vi "Conversion.vi"(0 "read buffer":string, 9 "Mechanical Zero":dbl) -> (3 "Static LF":dbl, 4 "Dynamic LF":dbl, 6 "Dynamic Load Force":dynamicdata(graph), 8 "Elbow Angle (deg)":dbl, 10 "GF":dbl, 13 "Static Load Force":dynamicdata(graph), 14 "Grip Force":dynamicdata(graph), 15 "Goniometer\nAngle Raw":dynamicdata(graph))   [LabVIEW 2018]
doc: "VI for GF and LF conversion."
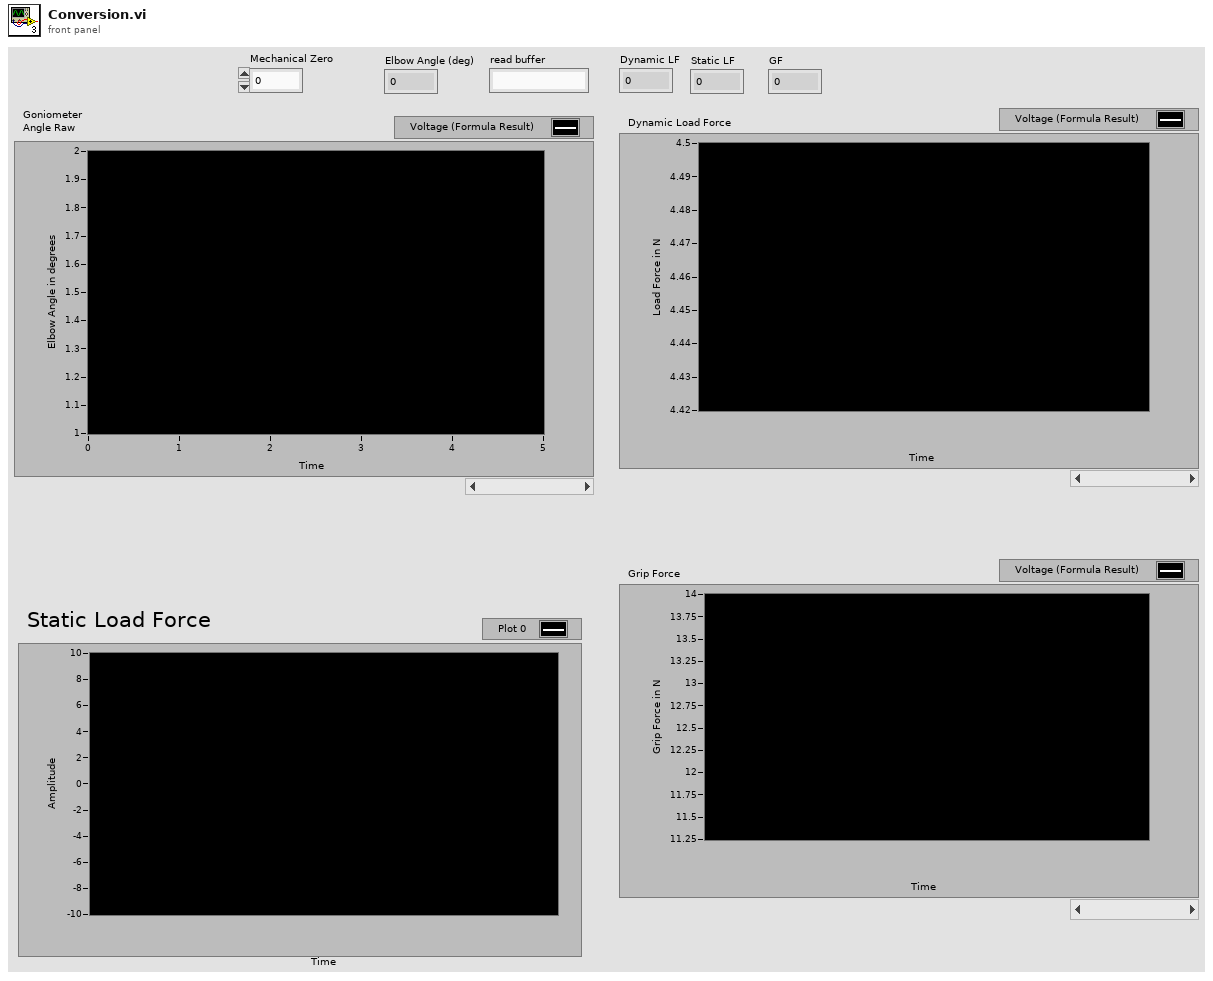
[diagram p1: front panel]
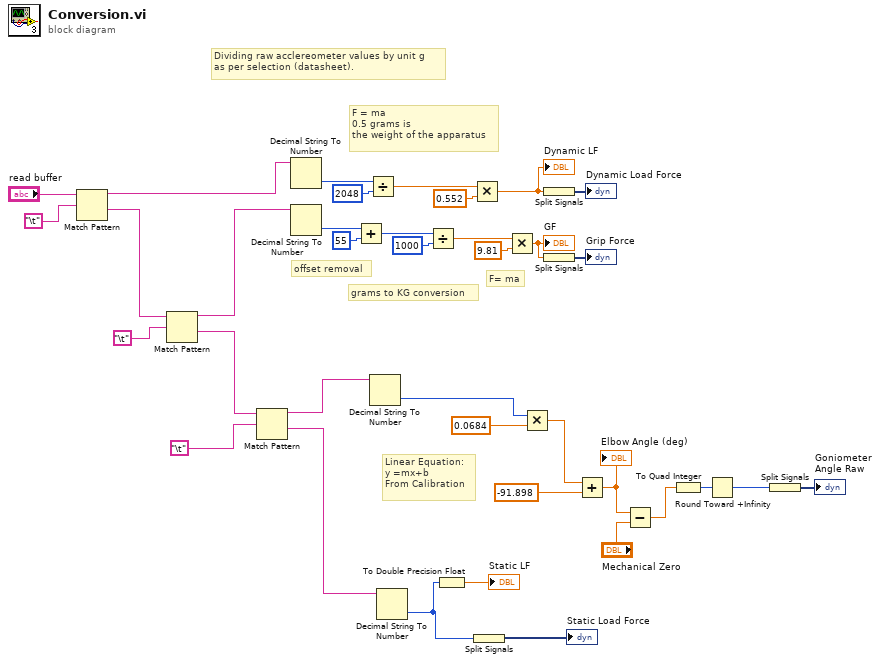
[diagram p0: block diagram]
diagram:
  # "Linear Equation:\ny =mx+b\nFrom Calibration"
  # "F= ma"
  # "offset removal"
  # "grams to KG conversion"
  # "F = ma\n0.5 grams is \nthe weight of the apparatus"
  # "Dividing raw acclereometer values by unit g\nas per selection (datasheet)."
  n1 = Match Pattern(string="read buffer", regular expression="\t") -> (before substring=w32:string, after substring=w19:string)  [unwired: 1 in, 2 out]
  n2 = Match Pattern(string=w19, regular expression="\t") -> (before substring=w18:string, after substring=w7:string)  [unwired: 1 in, 2 out]
  n3 = Match Pattern(string=w7, regular expression="\t") -> (before substring=w6:string, after substring=w5:string)  [unwired: 1 in, 2 out]
  n4 = Decimal String To Number(string=w32) -> (number=w26:i32)  [unwired: 2 in, 1 out]
  n5 = Decimal String To Number(string=w18) -> (number=w34:i32)  [unwired: 2 in, 1 out]
  n6 = Add(x=w34, y=55) -> (x+y=w36:i32)
  n7 = Divide(x=w26, y=2048) -> (x/y=w24:dbl)
  n8 = Decimal String To Number(string=w6) -> (number=w13:i32)  [unwired: 2 in, 1 out]
  n9 = Decimal String To Number(string=w5) -> (number=w3:i32)  [unwired: 2 in, 1 out]
  n10 = Divide(x=w36, y=1000) -> (x/y=w29:dbl)
  n11 = To Double Precision Float(number=w3) -> (double precision float=→"Static LF":dbl)
  n12 = Multiply(x=w24, y=0.552) -> (x*y=w23:dbl)
  "Dynamic LF" <- w23
  n13 = Split Signals(w3) -> (→"Static Load Force":dynamicdata)  [unwired: 1 in]
  n14 = Multiply(x=w29, y=9.81) -> (x*y=w37:dbl)
  "GF" <- w37
  n15 = Multiply(x=w13, y=0.0684 ("x")) -> (x*y=w16:dbl)
  n16 = Split Signals(w23) -> (→"Dynamic Load Force":dynamicdata)  [unwired: 1 in]
  n17 = Split Signals(w37) -> (→"Grip Force":dynamicdata)  [unwired: 1 in]
  n18 = Add(x=w16, y=-91.898 ("x")) -> (x+y=w11:dbl)
  "Elbow Angle (deg)" <- w11
  n19 = Subtract(x=w11, y="Mechanical Zero") -> (x-y=w12:dbl)
  n20 = To Quad Integer(1:w12) -> (0:w9:i64)
  n21 = Round Toward +Infinity(x=w9) -> (ceil(x): smallest int >= x=w8:i64)
  n22 = Split Signals(w8) -> (→"Goniometer\nAngle Raw":dynamicdata)  [unwired: 1 in]
